vi "Module Main.vi"(8 "error in (no error)":errorcluster) -> (0 "error out":errorcluster)   [LabVIEW 2020, in "User Console.lvlib"]
doc: "Module Main\nFor named purposes"
uses:
  User Console.lvlib
  Public Control/Elevator Call.ctl
  Public Control/Floor Selection.ctl
  Public Control/Door Button.ctl
  Private Control/Queue FGV Action.ctl
  Error/Error.lvlib
panel:
  in  "Emergency":bool
  in  "Door Button":T1
  in  "Floor Selection":T2
  in  "Elevator Call":T3
  # "User Console"
  # "Fourth Floor"
  # "Third  Floor"
  # "Second Floor"
  # "First Floor"
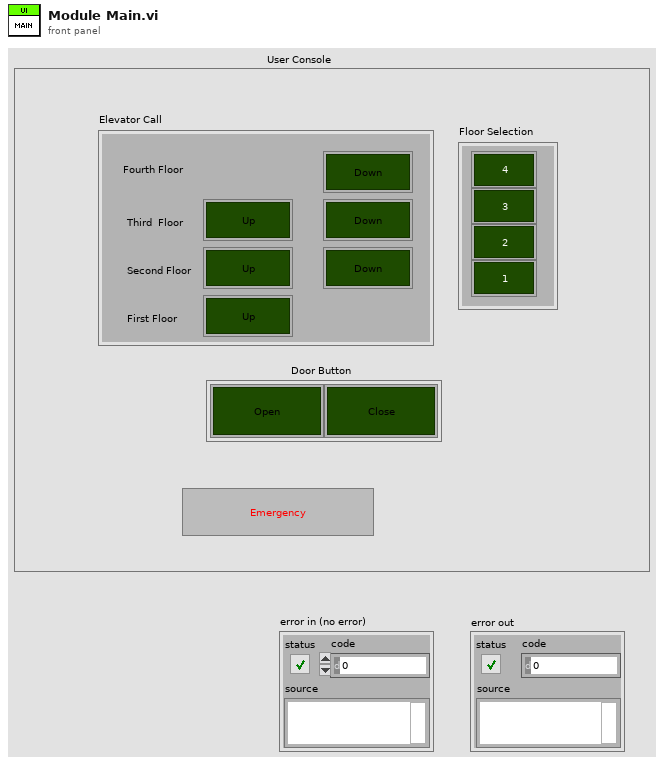
[diagram p1: front panel]
types:
  T1 = typedef "User Console.lvlib/Door Button.ctl" = cluster{"Open":bool, "Close":bool}
  T2 = typedef "User Console.lvlib/Floor Selection.ctl" = cluster{"4":bool, "3":bool, "2":bool, "1":bool}
  T3 = typedef "User Console.lvlib/Elevator Call.ctl" = cluster{"4_Down":bool, "3_Down":bool, "3_Up":bool, "2_Up":bool, "2_Down":bool, "1_Up":bool}
  T4 = typedef "User Console.lvlib/Queue FGV Action.ctl" = enum16{"Create", "Get", "Release"}
  T5 = typedef "User Console.lvlib/Queue Element.ctl" = cluster{"Module Action":T6, "Data":variant}
  T6 = typedef "User Console.lvlib/Module Action.ctl" = enum16{"Init", "Error", "Exit"}
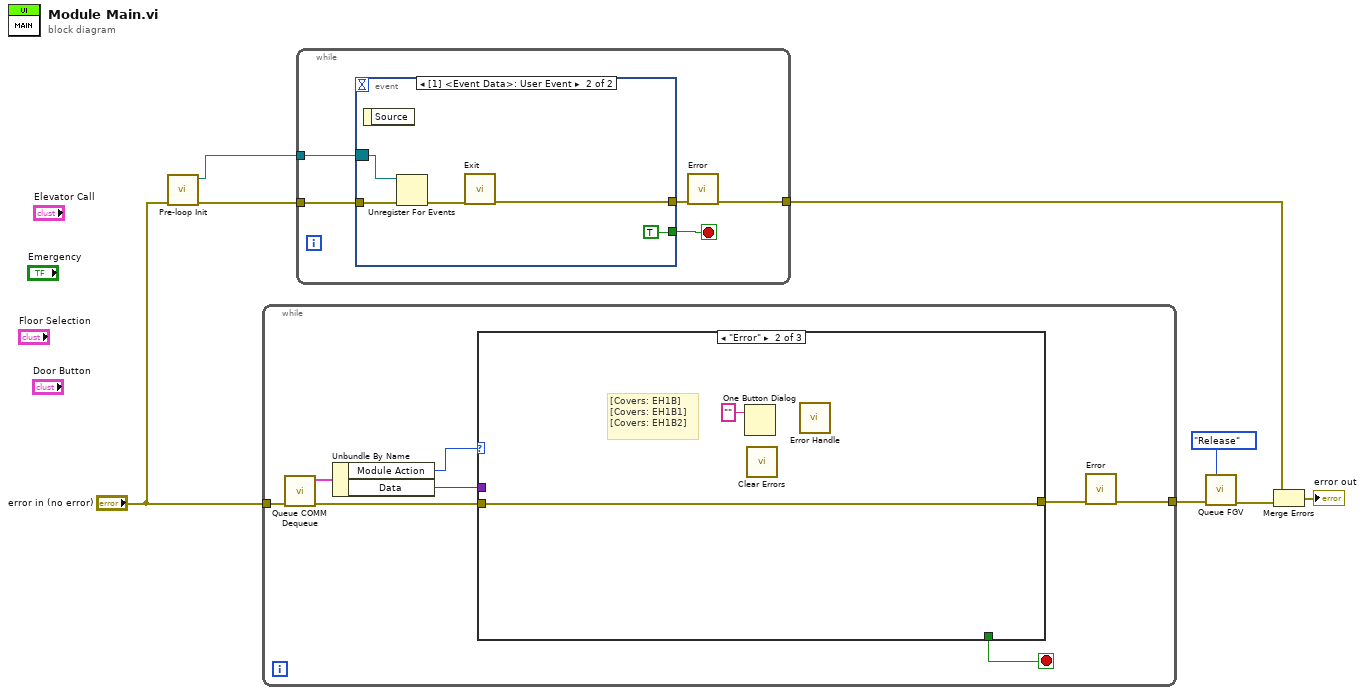
[diagram p0: block diagram]
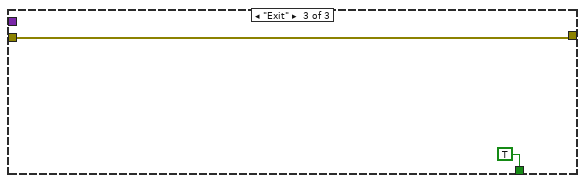
[diagram p3: hidden frame]
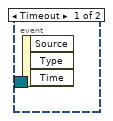
[diagram p4: hidden frame]
diagram:
  n1 = call "Pre-loop Init.vi"("error in (no error)"="error in (no error)") -> ("error out"=w7:errorcluster, "Event Registration Refnum"=w8:refnum<event-registration>)  [unwired: 9 in]
  n2 = while {
    tunnel: "error in (no error)" -> [w16]
    tunnel: [w10] -> w3
    stop <- w9 stop-if-true
    n3 = call "Queue COMM Dequeue.vi"("error in (no error)"=w16) -> ("error out"=w14:errorcluster, "element"=w15:T5)  [unwired: 9 in]
    n4 = Unbundle By Name(w15) -> ("Module Action"=w13:T6, "Data"=w12:variant)
    n5 = case shown="\"Error\"" w13 {
      tunnel: w14 -> [w17 w19 w21]
      tunnel: w12 -> [_ _ _]
      tunnel: [w17 w19 w21] -> w11
      tunnel: [_ _ TRUE] -> w9
      frame "Init", Default {
      }
      frame "Error" {
        # "[Covers: EH1B] \n[Covers: EH1B1] \n[Covers: EH1B2]"
        n6 = One Button Dialog(message="") -> ()  [unwired: 1 in, 1 out]
        n7 = call <vilib>:"Clear Errors.vi"() -> ()  [unwired: 6 in, 2 out]
        n8 = call "Error Handle.vi"() -> ()  [unwired: 11 in, 1 out]
      }
      frame "Exit" {
      }
    }
    n9 = call "Error.vi"("error in (no error)"=w11) -> ("error out"=w10:errorcluster)  [unwired: 10 in]
  }
  n10 = while {
    tunnel: w8 -> [w26]
    tunnel: w7 -> [w25]
    tunnel: [w23] -> w5
    stop <- w22 stop-if-true
    n11 = event shown="[1] <Event Data>: User Event" {
      selector: w26 -> [_ w30]
      dyn-events: _ -> [_ _]
      timeout: _ -> [_ _]
      tunnel: w25 -> [_ w31]
      tunnel: [_ w28] -> w24
      tunnel: [_ TRUE] -> w22
      event Timeout {
        n12 = event-data() -> ()  [unwired: 1 in, 3 out]
      }
      event User Event {
        n13 = event-data() -> ()  [unwired: 1 in, 1 out]
        n14 = Unregister For Events(event registration refnum=w30, error in=w31) -> (error out=w29:errorcluster)
        n15 = call "Exit.vi"("error in (no error)"=w29) -> ("error out"=w28:errorcluster)  [unwired: 10 in]
      }
    }
    n16 = call "Error.vi"("error in (no error)"=w24) -> ("error out"=w23:errorcluster)  [unwired: 10 in]
  }
  n17 = call "Queue FGV.vi"("error in (no error)"=w3, "Queue FGV  Action"=Queue_FGV_Action."Release") -> ("error out"=w2:errorcluster)  [unwired: 8 in, 1 out]
  n18 = Merge Errors(w5, w2) -> (→"error out":errorcluster)
